vi "Prober_ProbeTouchdown.vi"(8 "error in (no error)":errorcluster, 11 "VeloxTeslaProbestation in":refnum<class "VeloxTeslaProbestation.lvclass">) -> (0 "error out":errorcluster, 1 "previous Z [µm]":i32, 2 "Z [µm]":i32, 3 "VeloxTeslaProbestation out":refnum<class "VeloxTeslaProbestation.lvclass">)   [LabVIEW 2018, in "VeloxTeslaProbestation.lvclass"]
uses:
  VeloxTeslaProbestation.lvclass
  Desktop/Kvasnicka/test_labview_library/Integration_toolkit_library/CascadeProbestation.lvlib
panel:
  out "Response":string
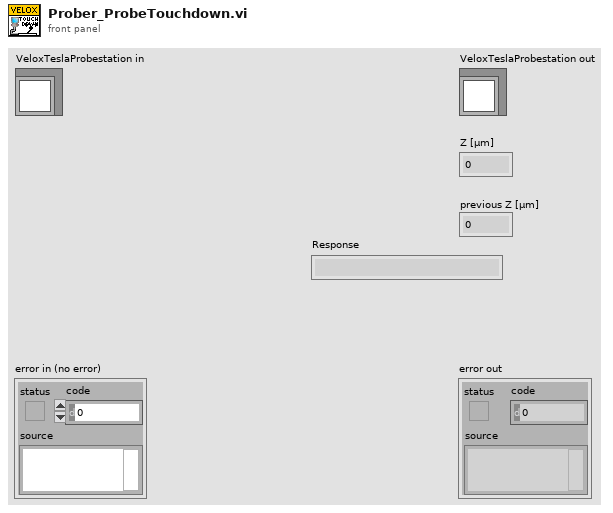
[diagram p1: front panel]
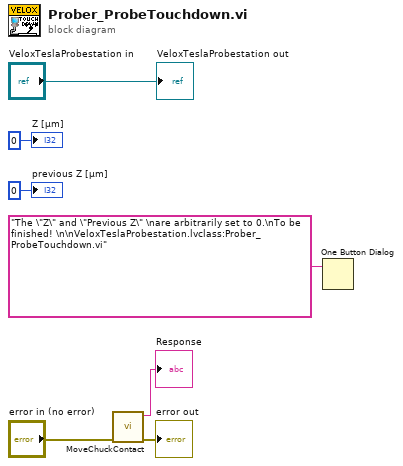
[diagram p0: block diagram]
diagram:
  n1 = call "MoveChuckContact.vi"("Error In"="error in (no error)") -> ("Error Out"=→"error out":errorcluster, "Response"=→"Response":string)  [unwired: 9 in]
  n2 = One Button Dialog(message="The \"Z\" and \"Previous Z\" \nare arbitrarily set to 0.\nTo be finished! \n\nVeloxTeslaProbestation.lvclass:Prober_ProbeTouchdown.vi") -> ()  [unwired: 1 in, 1 out]
  "VeloxTeslaProbestation out" <- "VeloxTeslaProbestation in"
  "previous Z [µm]" <- 0 ("previous Z [µm]")
  "Z [µm]" <- 0 ("Z [µm]")
